vi "file extension and new name.vi"(8 "error in":errorcluster, 10 "custom device name":string, 11 "filename":string) -> (0 "error out":errorcluster, 2 "extension":string, 3 "new filename":string)   [LabVIEW 2020, in "Template Tool.lvlib"]
uses:
  Template Tool.lvlib
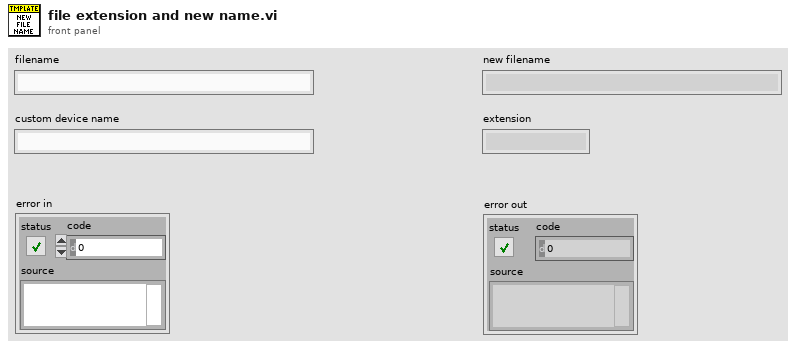
[diagram p1: front panel]
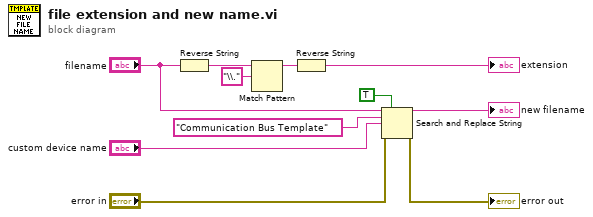
[diagram p0: block diagram]
diagram:
  n1 = Reverse String(1:"filename") -> (0:w9:string)
  n2 = Match Pattern(string=w9, regular expression="\\.") -> (before substring=w11:string)  [unwired: 1 in, 3 out]
  n3 = Reverse String(1:w11) -> (0:→"extension":string)
  n4 = Search and Replace String(replace all?=TRUE ("replace all? (F)"), input string="filename", search string="Communication Bus Template" ("regular expression"), replace string="custom device name", error in="error in") -> (result string=→"new filename":string, error out=→"error out":errorcluster)  [unwired: 3 in, 2 out]
